vi "Hardware-LEDs.vi"(0 "LoopPeriod [sec]":sgl, 5 "Activity Blink Rate [Hz]":sgl=1.0) -> (14 "User LED 1":T1, 15 "User LED 2":T1)   [LabVIEW 2016, in "DSI-RT.lvlib"]
uses:
  DSI-RT.lvlib
  <vilib>/Powertrain Controls/Device Drivers/DCM/Rev0/RT/User LED.ctl
  Shared/Typedefs/ErrorLEDState.ctl
  <vilib>/addons/Software Calibration Management/xSCM/FaultPoint.xnode
  <vilib>/Powertrain Controls/Device Drivers/DCM/Rev0/RT/DCM - RT.lvclass
  <vilib>/addons/Software Calibration Management/xSCM/ni_scm.dll
  Shared/DSI-Shared.lvlib
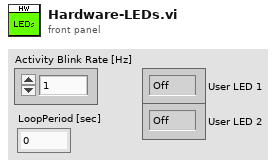
[diagram p1: front panel]
types:
  T1 = typedef "DCM - RT.lvclass/User LED.ctl" = enum16{"Off", "Yellow", "Green"}
  T2 = typedef "DSI-Shared.lvlib/ErrorLEDState.ctl" = enum16{"Idle", "Check Error", "Flashing", "Long Flash"}
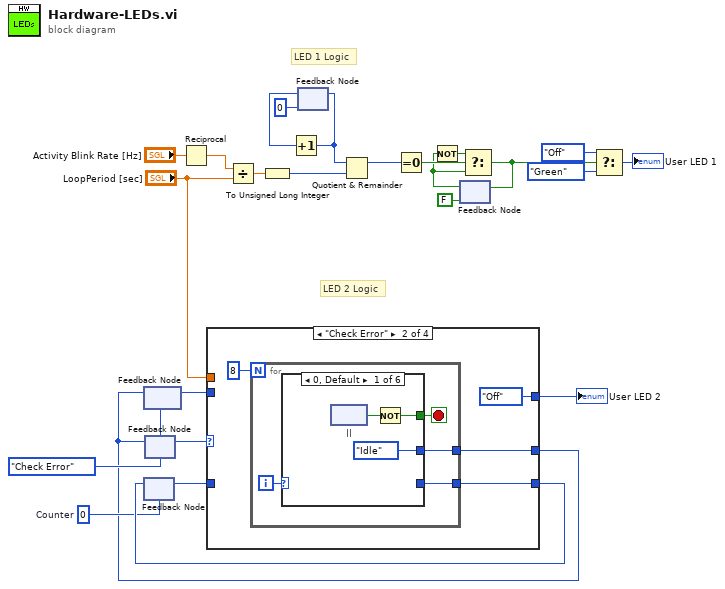
[diagram p0: block diagram]
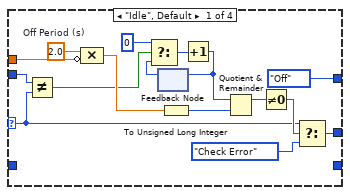
[diagram p2: hidden frame]
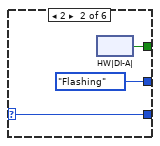
[diagram p3: hidden frame]
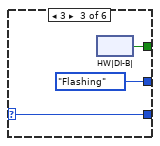
[diagram p4: hidden frame]
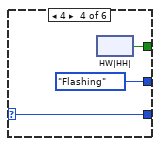
[diagram p5: hidden frame]
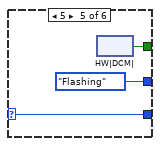
[diagram p6: hidden frame]
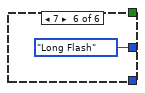
[diagram p7: hidden frame]
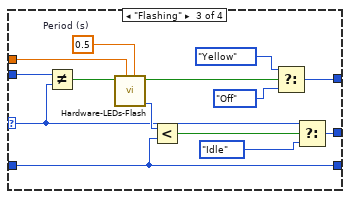
[diagram p8: hidden frame]
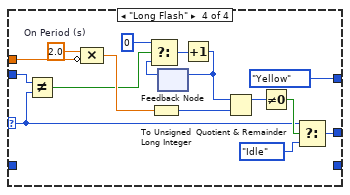
[diagram p9: hidden frame]
diagram:
  w5 = 0  # Counter
  w4 = ErrorLEDState."Check Error"
  # "LED 2 Logic"
  # "LED 1 Logic"
  n1 = feedback #1(w4) -> (w3:T2)
  n2 = feedback #2(w5) -> (w6:i32)
  n3 = feedback #3(w4) -> (w9:T2)
  n4 = Reciprocal(x="Activity Blink Rate [Hz]") -> (1/x=w1:sgl)
  n5 = case shown="\"Check Error\"" w9 {
    selector: w9 -> [w28 _ w88 w102]
    tunnel: [w41 w44 w99 w115] -> w2
    tunnel: [User_LED."Off" ("User LED 2") User_LED."Off" ("User LED 2") w97 User_LED."Yellow" ("User LED 2")] -> w10
    tunnel: "LoopPeriod [sec]" -> [w38 _ w93 w112]
    tunnel: [_ w43 w91 _] -> w7
    tunnel: w6 -> [_ _ w91 _]
    tunnel: w3 -> [w29 _ w87 w103]
    frame "Idle", Default {
      w39 = sgl 2.0  # Off Period (s)
      n6 = Not Equal?(x=w29, y=w28) -> (x != y?=w27:bool)
      n7 = Compound Arithmetic op=MULTIPLY(w39, invert w38) -> (w37:sgl)
      n8 = feedback #4() -> (w31:u32)  [unwired: 1 in]
      n9 = Select(t=u32 0, s=w27, f=w31) -> (s? t:f=w32:u32)
      n10 = To Unsigned Long Integer(number=w37) -> (unsigned 32bit integer=w26:u32)
      n11 = Increment(x=w32) -> (x+1=w36:u32)
      n12 = feedback-in #4(w36) -> ()
      n13 = Quotient & Remainder(x=w36, y=w26) -> (x-y*floor(x/y)=w35:u32)  [unwired: 1 out]
      n14 = Not Equal To 0?(x=w35) -> (x != 0?=w34:bool)
      n15 = Select(t=w28, s=w34, f=ErrorLEDState."Check Error") -> (s? t:f=w41:T2)
    }
    frame "Check Error" {
      # "Check Error State"
      n16 = for {
        N: 8 ("N Cases") -> [_]
        tunnel: [w47] -> w44
        tunnel: [w46] -> w43
        i -> [w49]
        stop <- w48 stop-if-true
        n17 = case shown="0, Default" w49 {
          selector: w49 -> [_ w57 w64 w71 w78 _]
          tunnel: [w50 w58 w65 w72 w79 _] -> w48
          tunnel: [ErrorLEDState."Idle" ErrorLEDState."Flashing" ErrorLEDState."Flashing" ErrorLEDState."Flashing" ErrorLEDState."Flashing" ErrorLEDState."Long Flash"] -> w47
          tunnel: [_ w57 w64 w71 w78 _] -> w46
          frame 0, Default {
            n18 = xnode "||"() -> ("Fault"=w51:bool)
            n19 = Not(x=w51) -> (.not. x?=w50:bool)
          }
          frame 2 {
            n20 = xnode "HW|DI-A|"() -> ("Fault"=w58:bool)
          }
          frame 3 {
            n21 = xnode "HW|DI-B|"() -> ("Fault"=w65:bool)
          }
          frame 4 {
            n22 = xnode "HW|HH|"() -> ("Fault"=w72:bool)
          }
          frame 5 {
            n23 = xnode "HW|DCM|"() -> ("Fault"=w79:bool)
          }
          frame 7 {
          }
        }
      }
    }
    frame "Flashing" {
      w89 = sgl 0.5  # Period (s)
      n24 = Not Equal?(x=w87, y=w88) -> (x != y?=w86:bool)
      n25 = call "Hardware-LEDs-Flash.vi"("Period (s)"=w89, "dt (s)"=w93, "Reset"=w86) -> ("Count"=w92:u32, "Output"=w95:bool)  [unwired: 7 in]
      n26 = Less?(x=w92, y=w91) -> (x < y?=w90:bool)
      n27 = Select(t=User_LED."Yellow" ("User LED 2"), s=w95, f=User_LED."Off" ("User LED 2")) -> (s? t:f=w97:T1)
      n28 = Select(t=w88, s=w90, f=ErrorLEDState."Idle") -> (s? t:f=w99:T2)
    }
    frame "Long Flash" {
      w113 = sgl 2.0  # On Period (s)
      n29 = Not Equal?(x=w103, y=w102) -> (x != y?=w101:bool)
      n30 = Compound Arithmetic op=MULTIPLY(w113, invert w112) -> (w111:sgl)
      n31 = To Unsigned Long Integer(number=w111) -> (unsigned 32bit integer=w100:u32)
      n32 = feedback #5() -> (w105:u32)  [unwired: 1 in]
      n33 = Select(t=u32 0, s=w101, f=w105) -> (s? t:f=w106:u32)
      n34 = Increment(x=w106) -> (x+1=w110:u32)
      n35 = feedback-in #5(w110) -> ()
      n36 = Quotient & Remainder(x=w110, y=w100) -> (x-y*floor(x/y)=w109:u32)  [unwired: 1 out]
      n37 = Not Equal To 0?(x=w109) -> (x != 0?=w108:bool)
      n38 = Select(t=w102, s=w108, f=ErrorLEDState."Idle") -> (s? t:f=w115:T2)
    }
  }
  "User LED 2" <- w10
  n39 = feedback-in #1(w2) -> ()
  n40 = feedback-in #2(w7) -> ()
  n41 = feedback-in #3(w2) -> ()
  n42 = Divide(x=w1, y="LoopPeriod [sec]") -> (x/y=w19:sgl)
  n43 = To Unsigned Long Integer(number=w19) -> (unsigned 32bit integer=w21:u32)
  n44 = feedback #6(u32 0) -> (w16:u32)
  n45 = Increment(x=w16) -> (x+1=w20:u32)
  n46 = feedback-in #6(w20) -> ()
  n47 = Quotient & Remainder(x=w20, y=w21) -> (x-y*floor(x/y)=w22:u32)  [unwired: 1 out]
  n48 = Equal To 0?(x=w22) -> (x = 0?=w15:bool)
  n49 = feedback #7(FALSE) -> (w12:bool)
  n50 = Not(x=w12) -> (.not. x?=w13:bool)
  n51 = Select(t=w13, s=w15, f=w12) -> (s? t:f=w11:bool)
  n52 = feedback-in #7(w11) -> ()
  n53 = Select(t=User_LED."Off" ("User LED 2"), s=w11, f=User_LED."Green" ("User LED 2")) -> (s? t:f=→"User LED 1":T1)
